vi "Send xyf move to stage.vi"(6 "Y move to send":sgl[unit], 8 "error in (no error)":errorcluster, 9 "X move to send":sgl[unit], 10 "focus move to send":dbl[unit], 11 "Retiga in":refnum<class "Retiga.lvclass">) -> (0 "error out":errorcluster, 3 "Retiga out":refnum<class "Retiga.lvclass">)   [LabVIEW 2012, in "Retiga.lvclass"]
uses:
  Retiga.lvclass
  <vilib>/Distrio/Murmex/GenericMessage/GenericMessage.lvclass
  Retiga.lvclass/Retiga.ctl
  <vilib>/Distrio/Murmex/Message/Message.lvclass
  <vilib>/Distrio/Murmex/Murmex/Murmex.lvclass
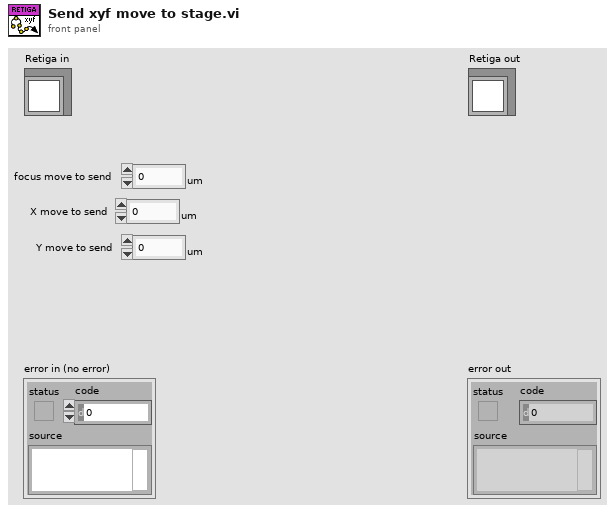
[diagram p1: front panel]
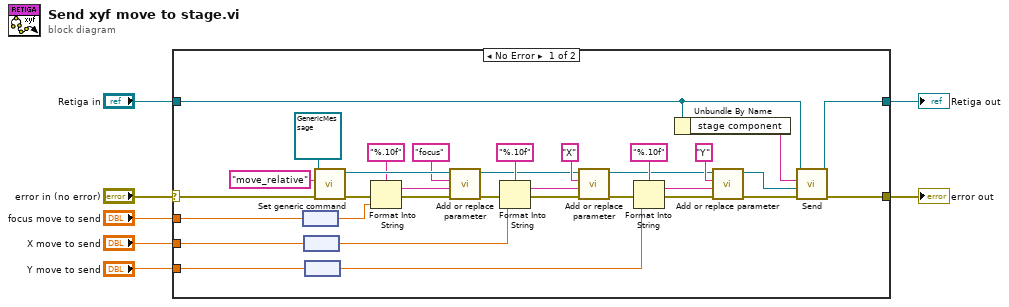
[diagram p0: block diagram]
diagram:
  n1 = case shown="No Error" "error in (no error)" {
    selector: "error in (no error)" -> [w31 w42]
    tunnel: [w30 w42] -> w6
    tunnel: [w28 w41] -> w4
    tunnel: "Retiga in" -> [w29 w41]
    tunnel: "focus move to send" -> [w27 _]
    tunnel: "X move to send" -> [w9 _]
    tunnel: "Y move to send" -> [w8 _]
    frame No Error {
      n2 = node(w27) -> (w12:dbl)
      n3 = node(w9) -> (w11:sgl)
      n4 = node(w8) -> (w10:sgl)
      n5 = call <vilib>:"Set generic command.vi"("error in (no error)"=w31, "generic command"="move_relative" ("command string"), "GenericMessage in"=refnum<class "GenericMessage.lvclass"> refnum ("Murmex.lvlib:GenericMessage")) -> ("error out"=w39:errorcluster, "GenericMessage out"=w40:refnum<class "GenericMessage.lvclass">)  [unwired: 7 in]
      n6 = Format Into String(format string="%.10f", error in=w39, w12) -> (resulting string=w37:string, error out=w38:errorcluster)  [unwired: 1 in]
      n7 = call <vilib>:"Add or replace parameter.vi"("error in (no error)"=w38, "value"=w37, "name"="focus", "Message in"=w40) -> ("error out"=w18:errorcluster, "Message out"=w16:refnum<class "GenericMessage.lvclass">)  [unwired: 6 in]
      n8 = Format Into String(format string="%.10f", error in=w18, w11) -> (resulting string=w25:string, error out=w26:errorcluster)  [unwired: 1 in]
      n9 = call <vilib>:"Add or replace parameter.vi"("error in (no error)"=w26, "value"=w25, "name"="X", "Message in"=w16) -> ("error out"=w17:errorcluster, "Message out"=w15:refnum<class "GenericMessage.lvclass">)  [unwired: 6 in]
      n10 = Format Into String(format string="%.10f", error in=w17, w10) -> (resulting string=w21:string, error out=w22:errorcluster)  [unwired: 1 in]
      n11 = Unbundle By Name(w29) -> ("stage component"=w33:string)
      n12 = call <vilib>:"Add or replace parameter.vi"("error in (no error)"=w22, "value"=w21, "name"="Y", "Message in"=w15) -> ("error out"=w13:errorcluster, "Message out"=w14:refnum<class "GenericMessage.lvclass">)  [unwired: 6 in]
      n13 = call <vilib>:"Send.vi"("error in (no error)"=w13, "Message"=w14, "recipient"=w33, "Murmex in"=w29) -> ("error out"=w30:errorcluster, "Murmex out"=w28:refnum<class "Retiga.lvclass">)  [unwired: 6 in]
    }
    frame Error {
    }
  }
  "error out" <- w6
  "Retiga out" <- w4
